vi "DeInterleave.vi"(7 "AlazarCluster":T1, 8 "Digitizer Settings":T5={"Digitizer delay (us) "=0.0, "rf points per line"=2048, "lines per plane"=128, "Samp Rate (Hz)"=100000000.0, "Additional dig delay (us)"=0.0, "Voltage Scale"=0.4, "Pre-Looks"=0, "Offset delay (us)"=0.0, "bits A/D"=8, "Avg Num"=1, "DigTimeOut"=5.0, "Rel Dig Delay"=0.0, "Dig Ch"=0, "LeCroyCluster"={"LeCroy Channels"=[TRUE, FALSE, FALSE, FALSE], "LC read pt offset"=0.0, "Sweep Avg"=FALSE}, "Main Digitizer"=enum."NI Digitizer", "Dig Config"=enum."Single channel", "Digitizer ID Cluster"={"Acqiris/Alazar/SP ID"=[], "NI Instr Handles"=[], "LeCroy VISA"="", "GaGe Handle"={"Handle"=0, "Sample size"=0, "Resolution"=0, "Offset"=0, "Channels"=0, "Boards"=0}, "ATS Ref"="ATS9350", "Acqiris Address"=["PCI::INSTR0"], "ADQRef"=refnum, "adq_cu_ptr"=refnum}, "Trigger Settings"={"Trig Source"=1, "Trig Coupling"=0, "Trig Slope"=0, "Level (mV)"=1500.0}, "Bulk Acq"=FALSE, "Bulk Start Indexes"=[], "Data Ref RF"=refnum, "NI ID/Channel"=[], "Total Dig CH"=1, "Xtra Ann Trig delay (us)"=10.0, "Fix Z Delay?"=FALSE, "One Way Transmission?"=FALSE, "Data Ref Log"=refnum} {"Trigger Settings"."Trig Slope" items=["Positive", "Negative"]; "Trigger Settings"."Level (mV)" format="%.2f"; "Trigger Settings"."Trig Coupling" items=["DC 1 MOhm", "AC 1 MOhm", "DC 50 Ohm", "AC 50 Ohm"]; "Trigger Settings"."Trig Source" items=["Chan 1", "External"]; "Rel Dig Delay" format="%.2f"; "DigTimeOut" format="%.2f"; "Avg Num" min=1; "Offset delay (us)" format="%.2f"; "Additional dig delay (us)" format="%.2f"; "Digitizer delay (us)" format="%.2f"}, 9 "Ann Array Params":T2={"Synth Foc?"=FALSE, "Focal Zones"=41, "Switch T/R"=0, "Trans Geometry (mm)"={"Transducer"=0, "Geo Focus"=12.0, "a (radius)"=3.0, "# of rings"=5, "kerf space "=0.1, "Center Freq"=12.0}, "Sub Ap Excite?"=FALSE, "Full Array Scan?"=FALSE, "Xmt/Rcv"={"XMIT"=[TRUE, TRUE, TRUE, TRUE, TRUE], "RCV"=[TRUE, TRUE, TRUE, TRUE, TRUE]}, "PulseSpacing (us)"=0.0, "Xmit Ring"=0, "XMIT CHS"=0, "RCV CHS"=0, "GPU?"=FALSE, "Save TIFF?"=FALSE, "downfactor"=1, "RCV 1CH"=0} {"RCV 1CH" items=["All", "1", "2", "3", "4", "5"]; "Trans Geometry (mm)"."Transducer" items=["6D 12R 40 MHz"=0, "10D 31R 20 MHz"=1, "10D 23R 20 MHz"=2, "6D 23R 40 MHz"=3, "4.5D 10.7R 40 MHz"=4, "9D 23.5R 20 MHz"=5, "9D 25.8R 20MHz"=6, "Enter"=99]; "Switch T/R" min=1 max=5 step=1}, 10 "Alazar Data":i16[](array[numeric]), 11 "Data in":i16[][](array[numeric]) caption="NI Data") -> (2 "Sorted Array Out":i16[](array[numeric]))   [LabVIEW 2022 SP3]
uses:
  ScanningControl/Digitizers/-DigitizerRoutines/DigitizerSettings.ctl
  ScanningControl/Digitizers/-DigitizerRoutines/Digitizer.ctl
  ScanningControl/Digitizers/-DigitizerRoutines/DigConfig.ctl
  ScanningControl/Digitizers/-DigitizerRoutines/DigitizerID.ctl
  C:/Windows/System32/ADQAPI_dotNet_helper.dll
  Annular Array/-AnnularRoutines/AnnularArray.ctl
  Annular Array/-AnnularRoutines/TransGeometry.ctl
  Annular Array/-AnnularRoutines/ArrayGeometry.ctl
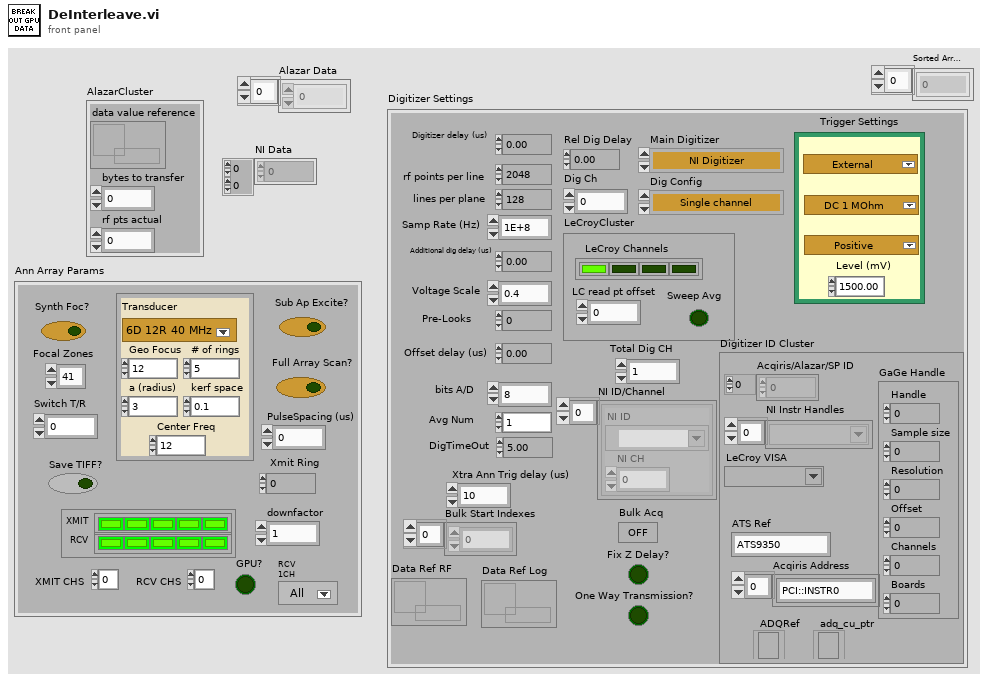
[diagram p1: front panel]
types:
  T1 = cluster{"data value reference":refnum<data-value>, "bytes to transfer":u32, "rf pts actual":u32}
  T2 = typedef "AnnularArray.ctl" = cluster{"Synth Foc?":bool, "Focal Zones":i16, "Switch T/R":i16, "Trans Geometry (mm)":T3, "Sub Ap Excite?":bool, "Full Array Scan?":bool, "Xmt/Rcv":cluster{"XMIT":bool[], "RCV":bool[]}, "PulseSpacing (us)":sgl, "Xmit Ring":i32, "XMIT CHS":u8, "RCV CHS":u8, "GPU?":bool, "Save TIFF?":bool, "downfactor":i32, "RCV 1CH":u16}
  T3 = typedef "TransGeometry.ctl" = cluster{"Transducer":T4, "Geo Focus":dbl, "a (radius)":dbl, "# of rings":i32, "kerf space ":dbl, "Center Freq":dbl}
  T4 = typedef "ArrayGeometry.ctl" = u16
  T5 = typedef "DigitizerSettings.ctl" = cluster{"Digitizer delay (us) ":dbl, "rf points per line":i32, "lines per plane":i32, "Samp Rate (Hz)":dbl, "Additional dig delay (us)":dbl, "Voltage Scale":dbl, "Pre-Looks":i32, "Offset delay (us)":dbl, "bits A/D":i8, "Avg Num":i32, "DigTimeOut":sgl, "Rel Dig Delay":sgl, "Dig Ch":i32, "LeCroyCluster":cluster{"LeCroy Channels":bool[], "LC read pt offset":dbl, "Sweep Avg":bool}, "Main Digitizer":T6, "Dig Config":T7, "Digitizer ID Cluster":T8, "Trigger Settings":cluster{"Trig Source":u16, "Trig Coupling":u16, "Trig Slope":u16, "Level (mV)":dbl}, "Bulk Acq":bool, "Bulk Start Indexes":i32[], "Data Ref RF":refnum<data-value>, "NI ID/Channel":cluster{"NI ID":refnum<k15>, "NI CH":i32}[], "Total Dig CH":i32, "Xtra Ann Trig delay (us)":dbl, "Fix Z Delay?":bool, "One Way Transmission?":bool, "Data Ref Log":refnum<data-value>}
  T6 = typedef "Digitizer.ctl" = enum16{"Acqiris Digitizer", "NI Digitizer", "LeCroy", "GaGe", "AlazarTech", "No Digitizer", "Teledyne"}
  T7 = typedef "DigConfig.ctl" = enum16{"Single channel", "2 Chans w/ 2 Acqiris", "2 Chans w/ 1 Acqiris", "5-CH Pulser New", "5-CH pulser w/ ann array", "5-pass style ann array", "Empty"}
  T8 = typedef "DigitizerID.ctl" = cluster{"Acqiris/Alazar/SP ID":u32[], "NI Instr Handles":refnum<k15>[], "LeCroy VISA":refnum<visa-resource-name>, "GaGe Handle":cluster{"Handle":u32, "Sample size":u32, "Resolution":i32, "Offset":i32, "Channels":u32, "Boards":u32}, "ATS Ref":string, "Acqiris Address":string[], "ADQRef":refnum<k24>, "adq_cu_ptr":refnum<k24>}
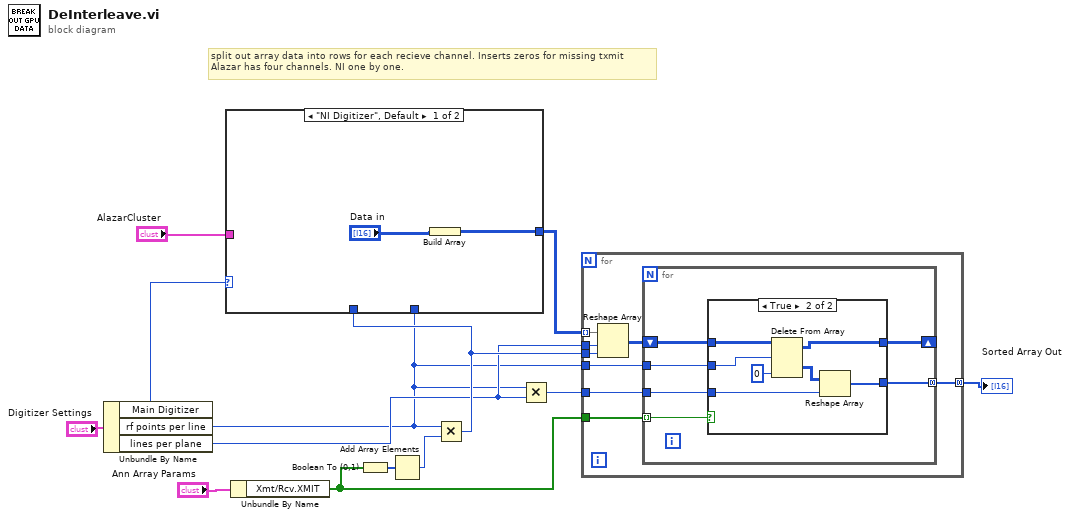
[diagram p0: block diagram]
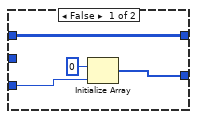
[diagram p2: hidden frame]
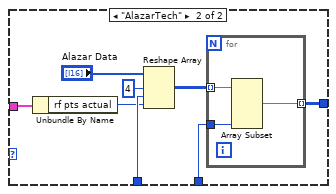
[diagram p3: hidden frame]
diagram:
  # "split out array data into rows for each recieve channel. Inserts zeros for missing txmit\nAlazar has four channels. NI one by one."
  n1 = Unbundle By Name("Digitizer Settings") -> ("Main Digitizer"=w7:T6, "rf points per line"=w2:i32, "lines per plane"=w3:i32)
  n2 = Unbundle By Name("Ann Array Params") -> ("Xmt/Rcv.XMIT"=w11:bool[])
  n3 = Boolean To (0,1)(Boolean=w11) -> (0, 1=w10:i16[])
  n4 = Add Array Elements(numeric array=w10) -> (sum=w1:i16)
  n5 = Multiply(x=w2, y=w1) -> (x*y=w5:i32)
  n6 = case shown="\"NI Digitizer\", Default" w7 {
    tunnel: [w15 w16] -> w13
    tunnel: w5 -> [_ w21]
    tunnel: "AlazarCluster" -> [_ w20]
    tunnel: w2 -> [_ w17]
    frame "NI Digitizer", Default {
      n7 = Build Array("Data in") -> (w15:i16[][][])
    }
    frame "AlazarTech" {
      n8 = Unbundle By Name(w20) -> ("rf pts actual"=w19:u32)
      n9 = Reshape Array("Alazar Data", 4 ("dimension size"), w21, w19) -> (w18:i16[][][])
      n10 = for {
        tunnel: w18 -> [w26] mode=indexing
        tunnel: w17 -> [w25]
        tunnel: [w24] -> w16 mode=indexing
        n11 = Array Subset(array=w26, length (col)=w25) -> (w24:i16[][])  [unwired: 3 in]
      }
    }
  }
  n12 = Multiply(x=w2, y=w3) -> (x*y=w8:i32)
  n13 = for {
    tunnel: w13 -> [w34] mode=indexing
    tunnel: w11 -> [w32]
    tunnel: [w31] -> w9 mode=concatenating
    tunnel: w3 -> [w28]
    tunnel: w8 -> [w30]
    tunnel: w5 -> [w27]
    tunnel: w2 -> [w29]
    n14 = Reshape Array(w34, w28, w27) -> (w33:i16[][])
    n15 = for {
      shift-right: [w36] -> _
      shift-left: w33 -> [w40]
      tunnel: w32 -> [w39] mode=indexing
      tunnel: [w38] -> w31 mode=concatenating
      tunnel: w29 -> [w37]
      tunnel: w30 -> [w35]
      n16 = case shown="True" w39 {
        tunnel: w40 -> [w43 w50]
        tunnel: [w44 w49] -> w38
        tunnel: w37 -> [_ w48]
        tunnel: [w43 w47] -> w36
        tunnel: w35 -> [w42 w46]
        frame False {
          n17 = Initialize Array(i8 0 ("element"), w42) -> (w44:i8[])
        }
        frame True {
          n18 = Delete From Array(array=w50, length=w48, index (col)=0 ("index (row)")) -> (deleted portion=w45:i16[][], array with subset deleted=w47:i16[][])  [unwired: 1 in]
          n19 = Reshape Array(w45, w46) -> (w49:i16[])
        }
      }
    }
  }
  "Sorted Array Out" <- w9
